vi "Authentication.vi"(7 "Need Authentication":bool, 8 "error in (no error)":errorcluster, 9 "Domain":string, 10 "Password":string, 11 "User name":string) -> (0 "error out":errorcluster, 1 "Domain 2":string, 2 "Password 2":string, 3 "User name 2":string, 5 "Need Authentication 2":bool)   [LabVIEW 2017, in "WebServiceImporter.lvlib" / "Main Panel.lvlib" / "Input WSDL.lvlib"]
uses:
  <vilib>/Platform/WebService/Main Panel/Pages/Input WSDL/Input WSDL.lvlib
panel:
  in  "Tab Control":enum32{"Page 1", "Page 2"}(tab)
  in  "Cancel":bool
  in  "OK":bool
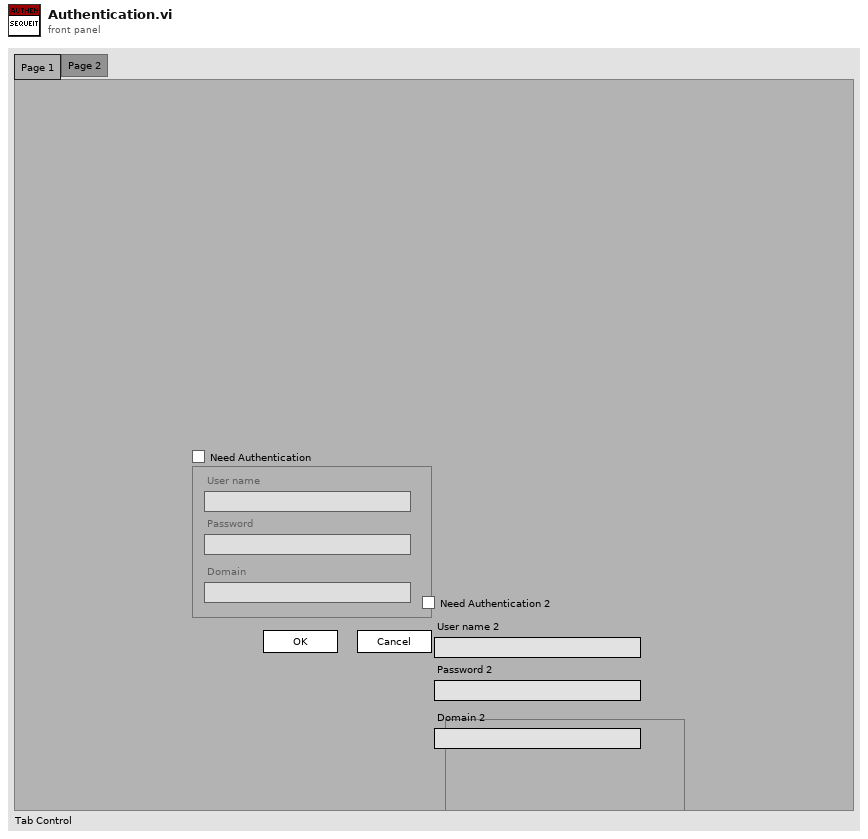
[diagram p1: front panel]
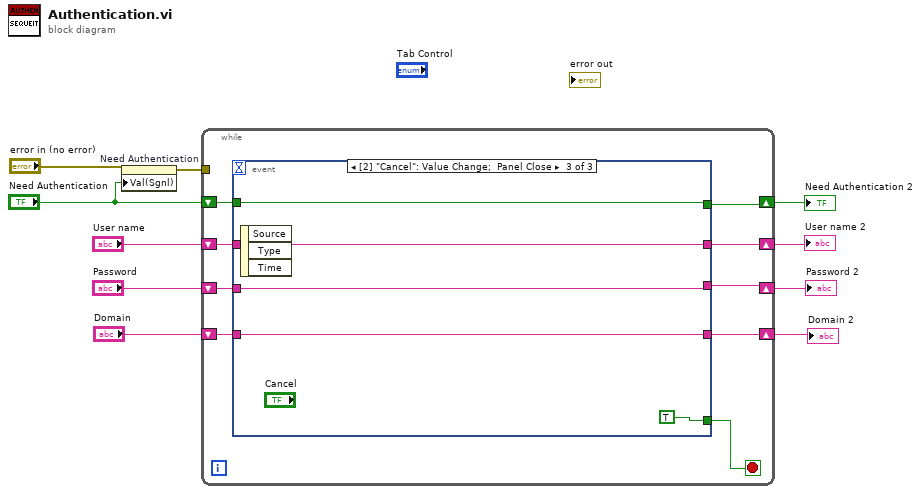
[diagram p0: block diagram]
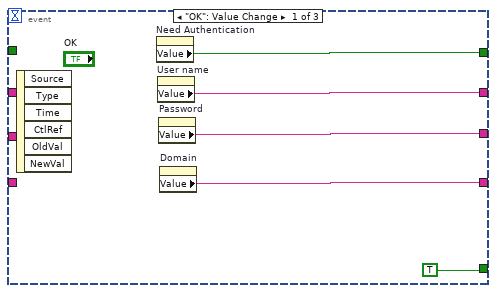
[diagram p2: hidden frame]
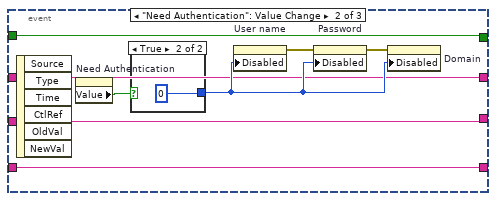
[diagram p3: hidden frame]
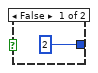
[diagram p4: hidden frame]
diagram:
  n1 = property on="Need Authentication" class="Bool (strict)"(error in="error in (no error)", "Val(Sgnl)"="Need Authentication") -> (error out=w2:errorcluster)  [unwired: 1 in, 1 out]
  n2 = while {
    shift-right: [w14] -> w7
    shift-left: "Need Authentication" -> [w15]
    shift-right: [w13] -> w6
    shift-left: "User name" -> [w18]
    shift-right: [w12] -> w5
    shift-left: "Password" -> [w17]
    shift-right: [w11] -> w4
    shift-left: "Domain" -> [w16]
    tunnel: w2 -> [_]
    stop <- w19 stop-if-true
    n3 = event shown="[2] \"Cancel\": Value Change;  Panel Close" {
      selector: _ -> [_ _ _]
      dyn-events: _ -> [_ _ _]
      timeout: _ -> [_ _ _]
      tunnel: [TRUE _ TRUE] -> w19
      tunnel: w18 -> [_ w27 w37]
      tunnel: w17 -> [_ w26 w36]
      tunnel: w16 -> [_ w25 w35]
      tunnel: w15 -> [_ w28 w38]
      tunnel: [w23 w28 w38] -> w14
      tunnel: [w22 w27 w37] -> w13
      tunnel: [w21 w26 w36] -> w12
      tunnel: [w20 w25 w35] -> w11
      event "OK": Value Change {
        n4 = event-data() -> ()  [unwired: 1 in, 6 out]
        n5 = property on="Need Authentication" class="Bool (strict)"() -> ("Value"=w23:bool)  [unwired: 2 in, 2 out]
        n6 = property on="User name" class="Str"() -> ("Value"=w22:string)  [unwired: 2 in, 2 out]
        n7 = property on="Password" class="Str"() -> ("Value"=w21:string)  [unwired: 2 in, 2 out]
        n8 = property on="Domain" class="Str"() -> ("Value"=w20:string)  [unwired: 2 in, 2 out]
      }
      event "Need Authentication": Value Change {
        n9 = event-data() -> ()  [unwired: 1 in, 6 out]
        n10 = property on="Need Authentication" class="Bool (strict)"() -> ("Value"=w29:bool)  [unwired: 2 in, 2 out]
        n11 = case shown="True" w29 {
          tunnel: [2 0] -> w30
          frame False {
          }
          frame True {
          }
        }
        n12 = property on="User name" class="Str"("Disabled"=w30) -> (error out=w32:errorcluster)  [unwired: 2 in, 1 out]
        n13 = property on="Password" class="Str"(error in=w32, "Disabled"=w30) -> (error out=w31:errorcluster)  [unwired: 1 in, 1 out]
        n14 = property on="Domain" class="Str"(error in=w31, "Disabled"=w30) -> ()  [unwired: 1 in, 2 out]
      }
      event "Cancel": Value Change; Panel Close {
        n15 = event-data() -> ()  [unwired: 1 in, 3 out]
      }
    }
  }
  "Need Authentication 2" <- w7
  "User name 2" <- w6
  "Password 2" <- w5
  "Domain 2" <- w4
